vi "Module_UI_TopLevel.vi"(8 "error in (no error)":errorcluster, 10 "Wait on Module(s) (\"\": none)":string) -> (0 "error out":errorcluster)   [LabVIEW 2020, in "Module_UI_TopLevel.lvclass"]
doc: "created using\nJSMA Module Template - UI Class 0.3.0.13\nRob Humfeld - Jet Engineering\nCopyright (c) 2020, Jet Engineering"
uses:
  Module_UI_TopLevel.lvclass
  Module_UI_TopLevel.lvclass/Module_UI_TopLevel.ctl
  <userlib>/JET Engineering/JET_QSM/Code/Private/JET_QSM - Add State to Front [String API].vi
  Private/Module_UI_TopLevel_jMsgTxList STYP.ctl
  <userlib>/JET Engineering/JET_QSM/Code/Private/JET_QSM - Add State [String API].vi
  Private/Module_UI_TopLevel_jMsgRxList STYP.ctl
  Private/Module_UI_TopLevel_LocalData STYP.ctl
  <userlib>/JET Labs/JET Panel/JETPanel.lvclass
  <userlib>/JET Engineering/JSMA/Libraries/jMsg_CORE/jMsg_JSMA_ApplicationShutdown/jMsg_JSMA_ApplicationShutdown.lvclass
  <userlib>/JET Engineering/JSMA/Libraries/jModule Class/jModule.lvclass
  <userlib>/JET Engineering/JSMA Standard Messages/jMsg_Sys_UIPanelOpen/jMsg_Sys_UIPanel_Open.lvclass
  shared/IPayable/IPayable.lvclass
  shared/AAccount/AAccount.lvclass
  <userlib>/Jet Labs/JET UITable/UITable.lvclass
  shared/IInfoable/IInfoable.lvclass
  Shared/Account Information STYP.ctl
  Account Types STYP.ctl
  C:/Program Files/National Instruments/LabVIEW 2020/user.lib/JET Engineering/JSMA/Libraries/jModule Class/jModule.lvclass
  C:/projects/budget_LabVIEW/Main Codeline/Software/Code/Module_UI_TopLevel/Module_UI_TopLevel.lvclass
  shared/SimpleChecking/SimpleChecking.lvclass
  shared/SimpleSavings/SimpleSavings.lvclass
  shared/SimpleCredit/SimpleCredit.lvclass
  C:/Program Files/National Instruments/LabVIEW 2020/user.lib/JET Engineering/JSMA/Libraries/jMsg Class/jMsg.lvclass
  C:/Program Files/National Instruments/LabVIEW 2020/user.lib/JET Engineering/JSMA Standard Messages/jMsg_Sys_UIPanelOpen/jMsg_Sys_UIPanel_Open.lvclass
  C:/Program Files/National Instruments/LabVIEW 2020/user.lib/JET Engineering/JSMA/Libraries/jMsg_CORE/jMsg_JSMA_ApplicationShutdown/jMsg_JSMA_ApplicationShutdown.lvclass
  C:/projects/budget_LabVIEW/Main Codeline/Software/Code/shared/ASavings/ASavings.lvclass
  C:/projects/budget_LabVIEW/Main Codeline/Software/Code/shared/AInterestAccount/AInterestAccount.lvclass
  C:/projects/budget_LabVIEW/Main Codeline/Software/Code/shared/AAccount/AAccount.lvclass
  C:/projects/budget_LabVIEW/Main Codeline/Software/Code/shared/IInfoable/IInfoable.lvclass
  C:/projects/budget_LabVIEW/Main Codeline/Software/Code/shared/IInterest/IInterest.lvclass
  C:/projects/budget_LabVIEW/Main Codeline/Software/Code/Shared/IDepositable/IDepositable.lvclass
  C:/projects/budget_LabVIEW/Main Codeline/Software/Code/shared/IWithdrawable/IWithdrawable.lvclass
  C:/projects/budget_LabVIEW/Main Codeline/Software/Code/shared/SimpleSavings/SimpleSavings.lvclass
  C:/projects/budget_LabVIEW/Main Codeline/Software/Code/shared/AChecking/AChecking.lvclass
  C:/projects/budget_LabVIEW/Main Codeline/Software/Code/shared/SimpleChecking/SimpleChecking.lvclass
  C:/projects/budget_LabVIEW/Main Codeline/Software/Code/shared/ACreditAccount/ACreditAccount.lvclass
  C:/projects/budget_LabVIEW/Main Codeline/Software/Code/shared/IBorrowable/IBorrowable.lvclass
  C:/projects/budget_LabVIEW/Main Codeline/Software/Code/shared/IPayable/IPayable.lvclass
  C:/projects/budget_LabVIEW/Main Codeline/Software/Code/shared/SimpleCredit/SimpleCredit.lvclass
panel:
  in  "Exit Button":bool
  in  "Expenses Button":bool
  in  "Accounts Button":bool
  in  "SubPanel":enum32{"Accounts", "Expenses", "Create Account"}(tab)
  in  "Remove Account Button":bool
  in  "Add Account Button":bool
  in  "Accounts List":i32(listbox)
  in  "Create Account Button":bool
  in  "Credit Limit Interval (s)":u32
  in  "Credit Limit":dbl
  in  "Account Type":T1
  in  "Routing Number":string
  in  "Initial Balance":dbl
  in  "Interest Interval (s)":u32
  in  "Interest Rate":dbl
  in  "Account Number":string
  out "winSizer B":string="W"
  out "winSizer A":string="W"
  out "jModule Name":string
  out "Recent states before Error (with tick counts) 2":string="0.167 sec ago: VI Initialize\n0.167 sec ago: Window Open\n0.110 sec ago: Control Update\n0.110 sec ago: Indicator Update\n0.000 sec ago: Error Handler\r\n"
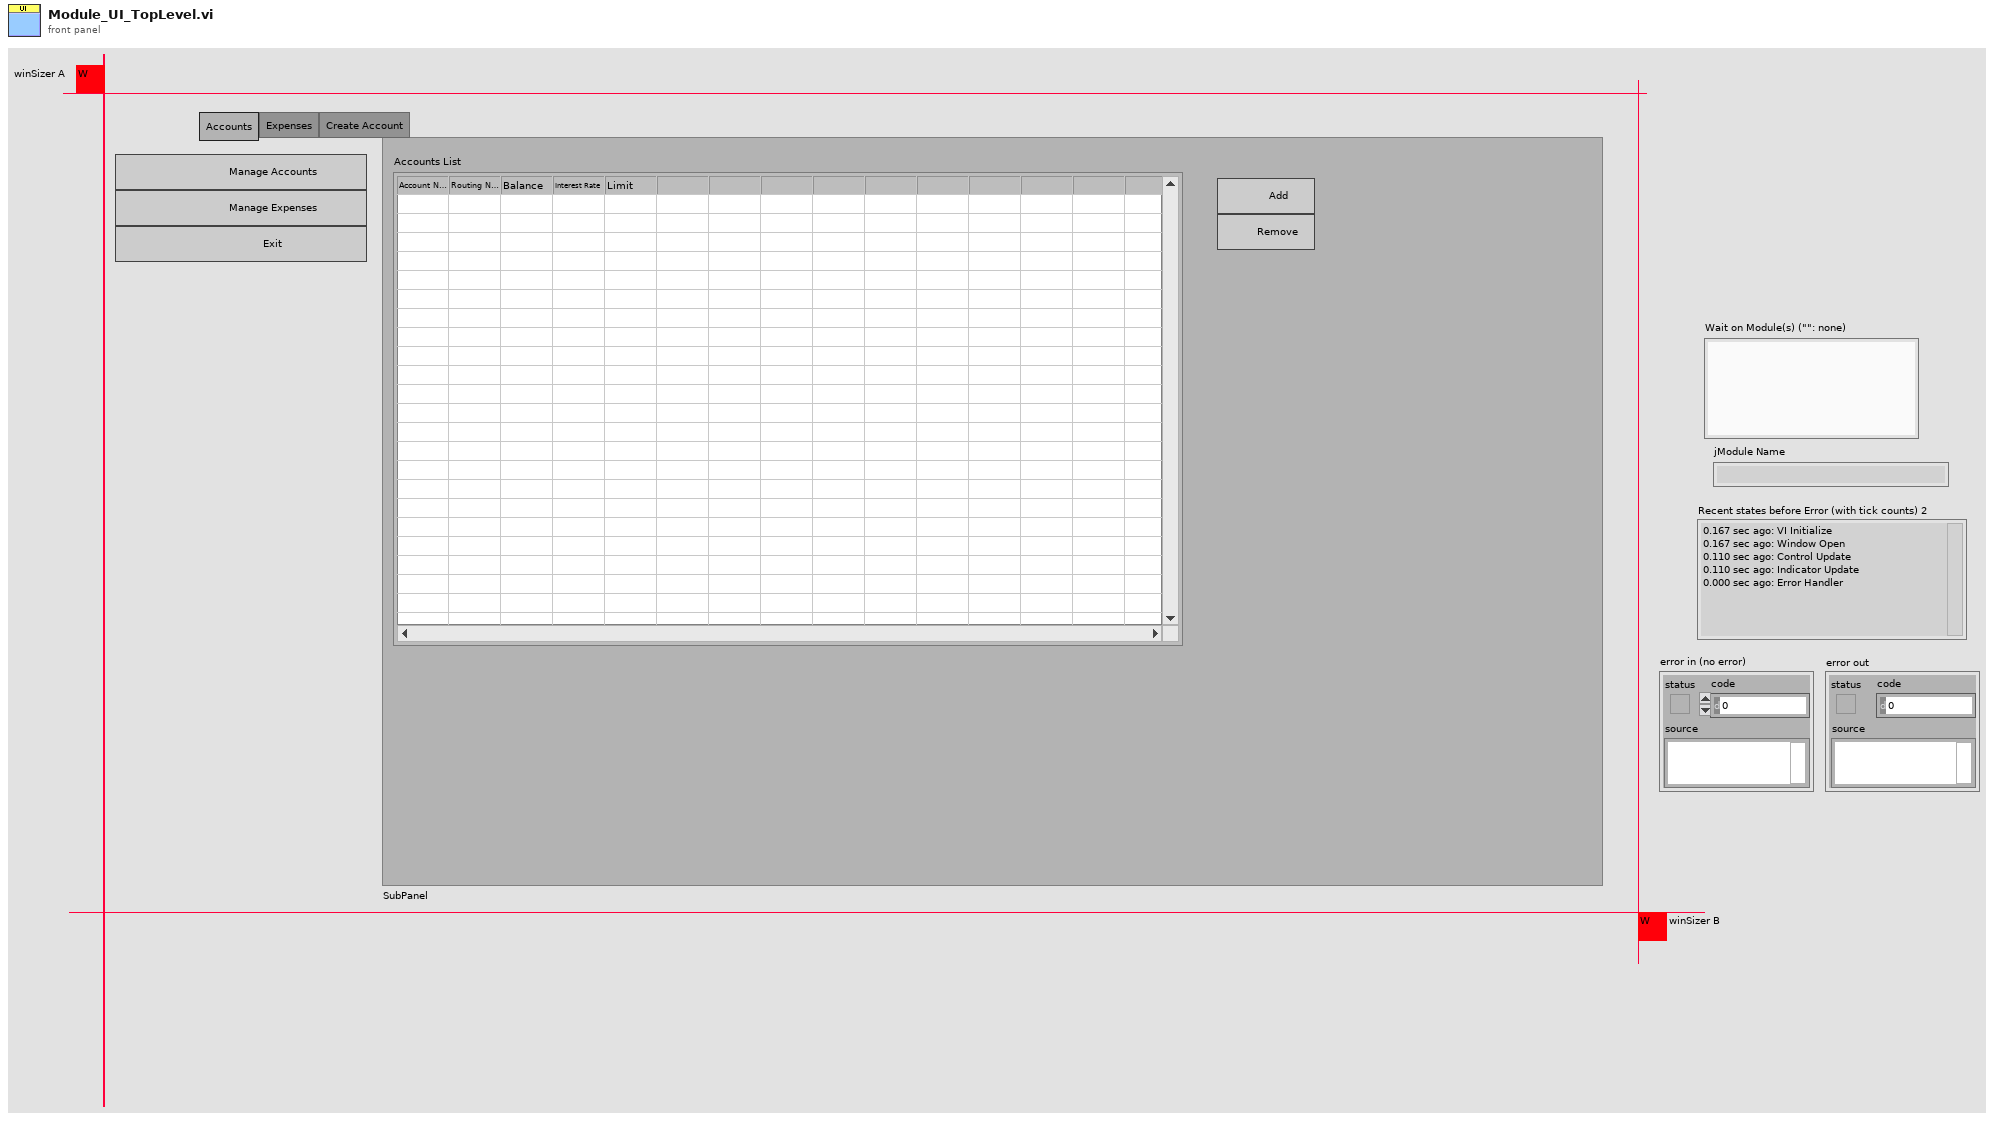
[diagram p1: front panel]
types:
  T1 = typedef "Module_UI_TopLevel.lvclass/Account Types STYP.ctl" = enum16{"Savings", "Checking", "Credit"}
  T2 = typedef "Module_UI_TopLevel.lvclass/Module_UI_TopLevel_LocalData STYP.ctl" = cluster{"VI":cluster{"error":errorcluster, "isExiting?":bool}, "UI":cluster{"Expenses":refnum<class "UITable.lvclass">, "Accounts Page":cluster{"Accounts":refnum<class "UITable.lvclass">, "Account Information":T3, "Interest Interval":u32, "Account Type":T1, "Credit Interval":u32}}, "Accounts":cluster{"Accounts":refnum<class "AAccount.lvclass">[]}, "Expenses":cluster{"Expenses":refnum<class "IPayable.lvclass">[]}}
  T3 = typedef "IInfoable.lvclass/Account Information STYP.ctl" = cluster{"Account Number":string, "Routing Number":string, "Balance":dbl, "Interest Rate":dbl, "Limit":dbl}
  T4 = typedef "Module_UI_TopLevel.lvclass/Module_UI_TopLevel_jMsgTxList STYP.ctl" = cluster{"jMsg_JSMA_ApplicationShutdown":refnum<class "jMsg_JSMA_ApplicationShutdown.lvclass">}
  T5 = typedef "Module_UI_TopLevel.lvclass/Module_UI_TopLevel_jMsgRxList STYP.ctl" = cluster{"jMsg_Sys_UIPanel_Open":refnum<class "jMsg_Sys_UIPanel_Open.lvclass">}
  T6 = typedef "JET_QSM_Refnum STYP.ctl" = cluster{"state":cluster{"queue":refnum<queue>, "idle":string, "error":string, "STOP":string}, "debug":cluster{"enabled?":bool, "queue":refnum<queue>}, "Invalid.option":T7, "QSM.Name":string}
  T7 = typedef "JET_QSM_InvalidOption STYP.ctl" = enum16{"Ignore", "Dialog", "Error"}
  T8 = typedef "JET_QSM_Element STYP.ctl" = cluster{"state":string, "data":variant, "comment":string}
  T9 = enum8{"Enabled", "Disabled", "Disabled and Grayed Out"}
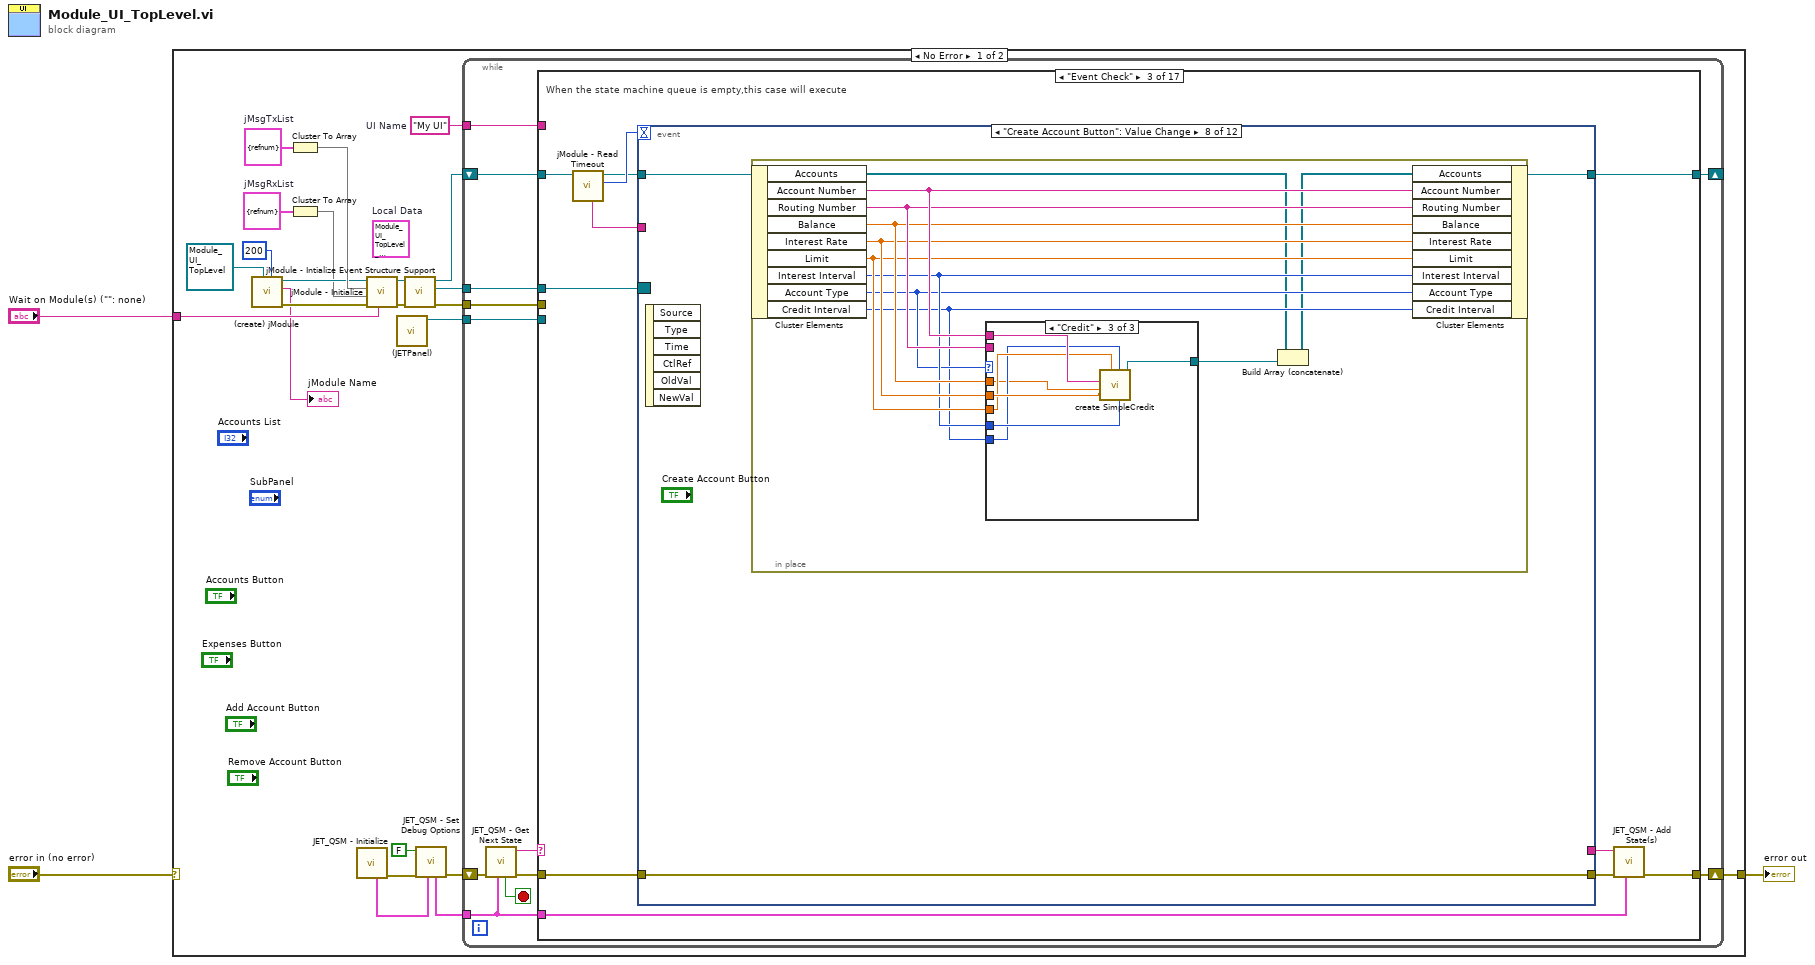
[diagram p0: block diagram]
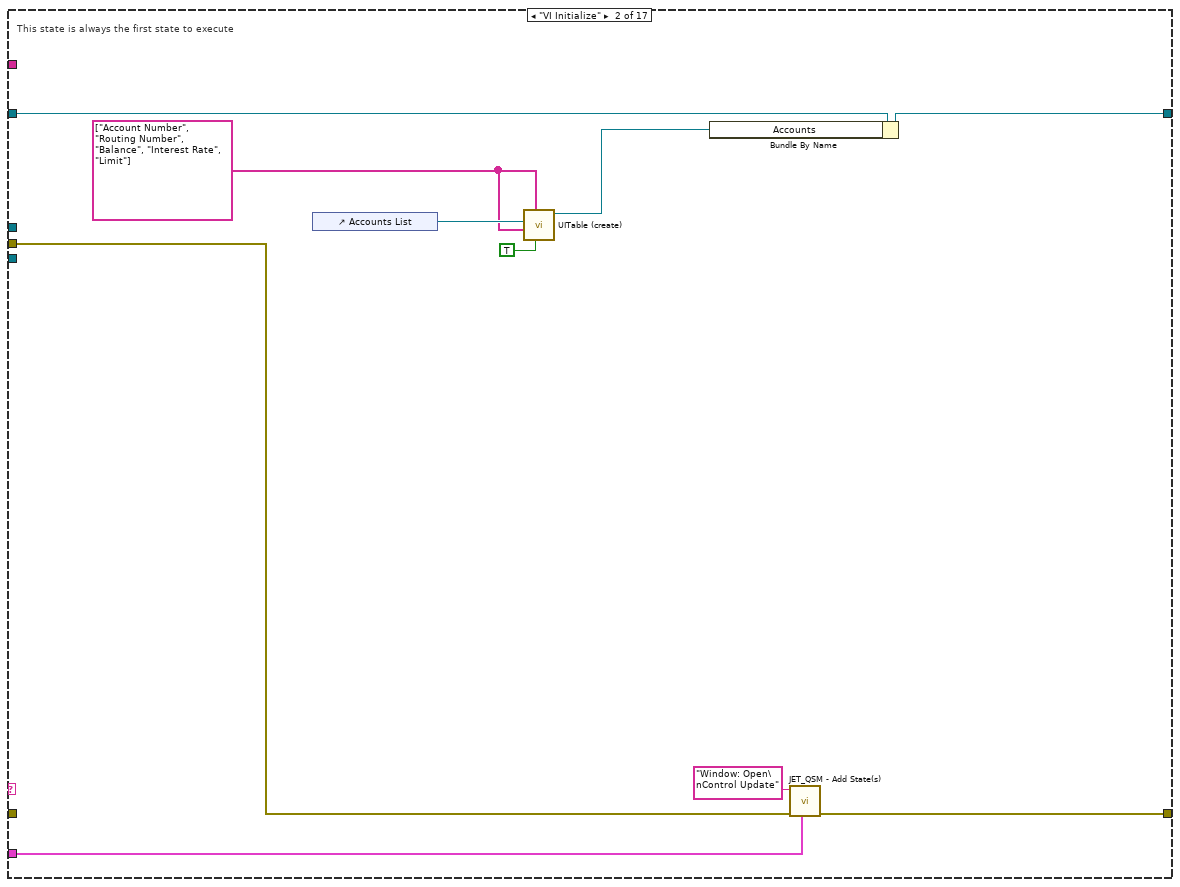
[diagram p3: hidden frame]
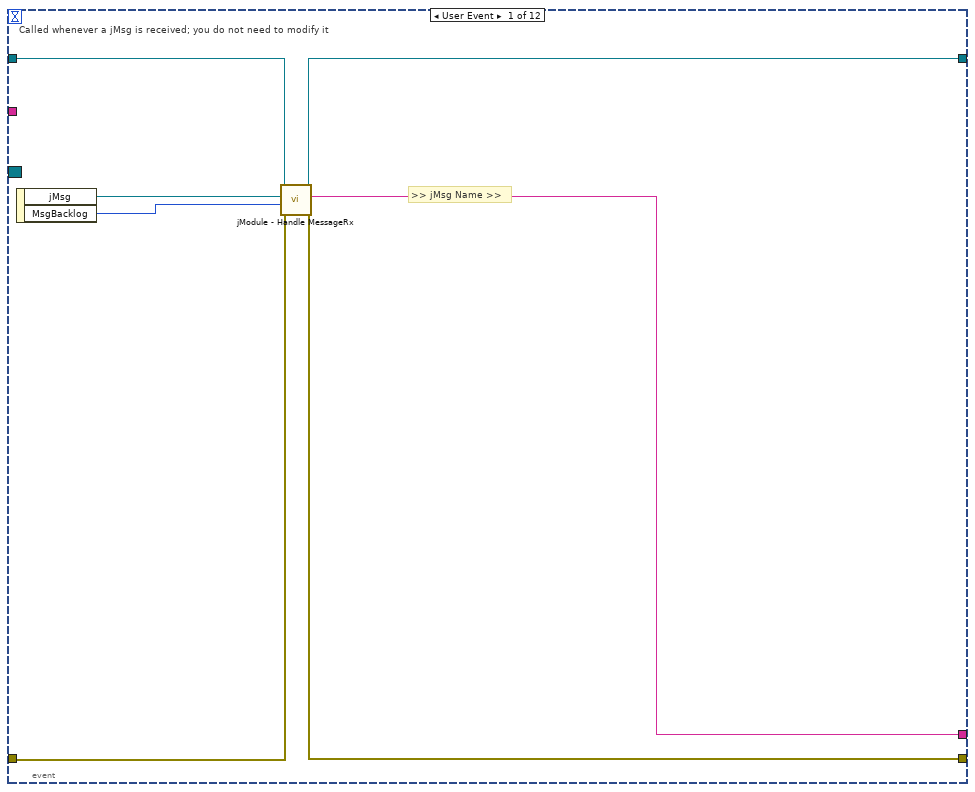
[diagram p4: hidden frame]
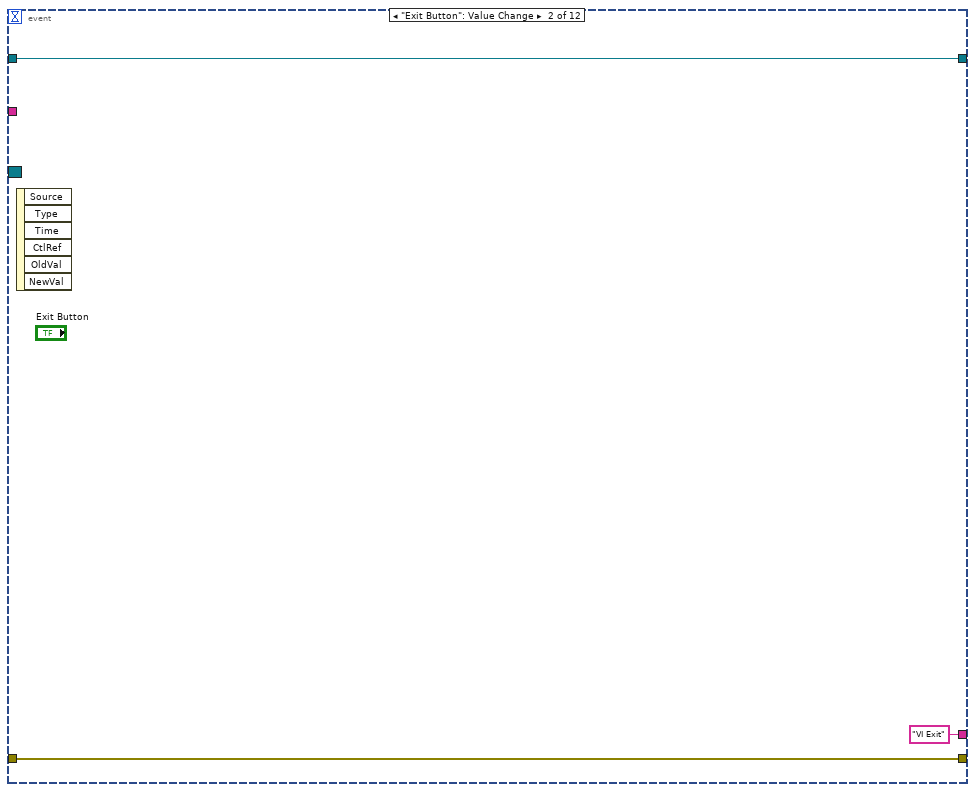
[diagram p5: hidden frame]
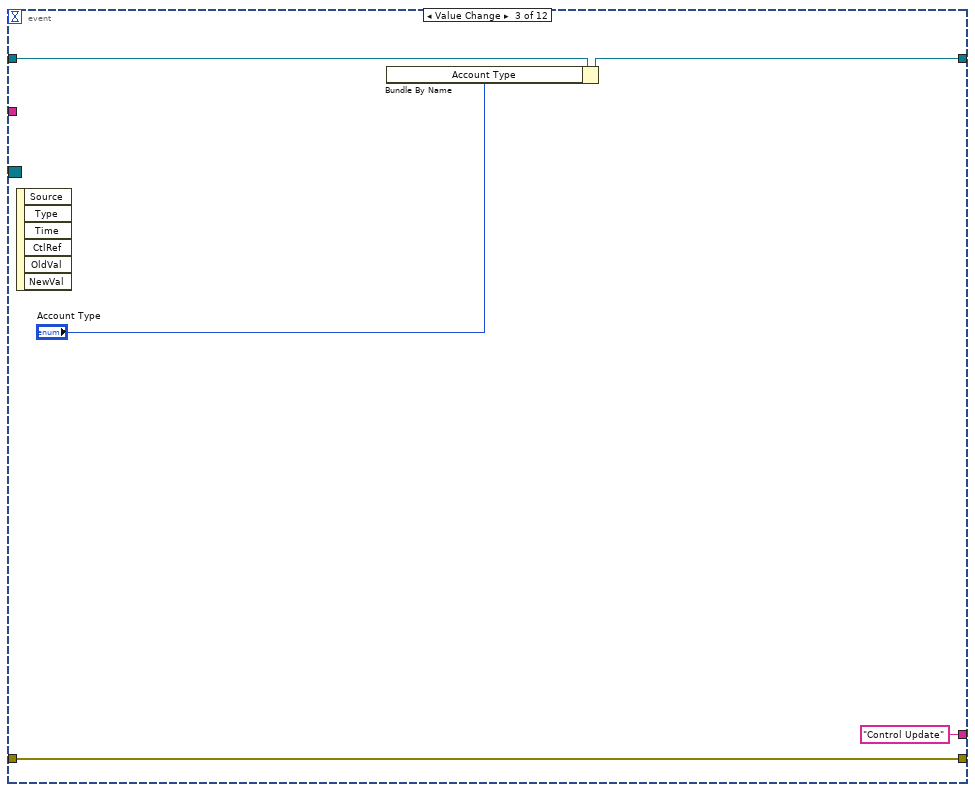
[diagram p6: hidden frame]
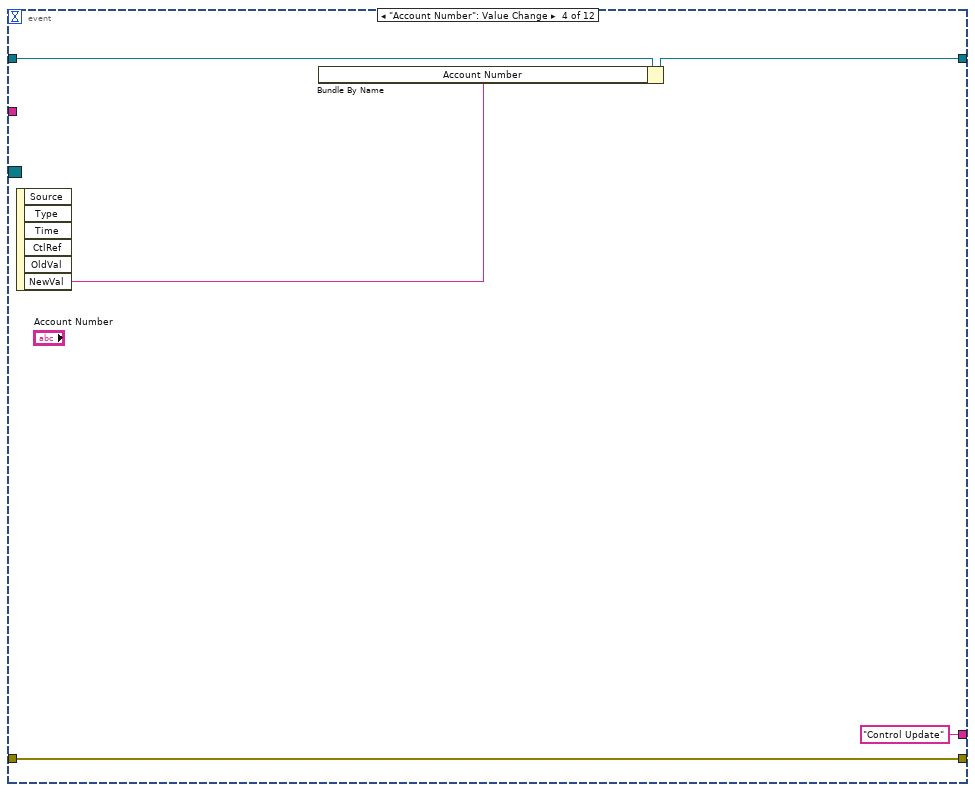
[diagram p7: hidden frame]
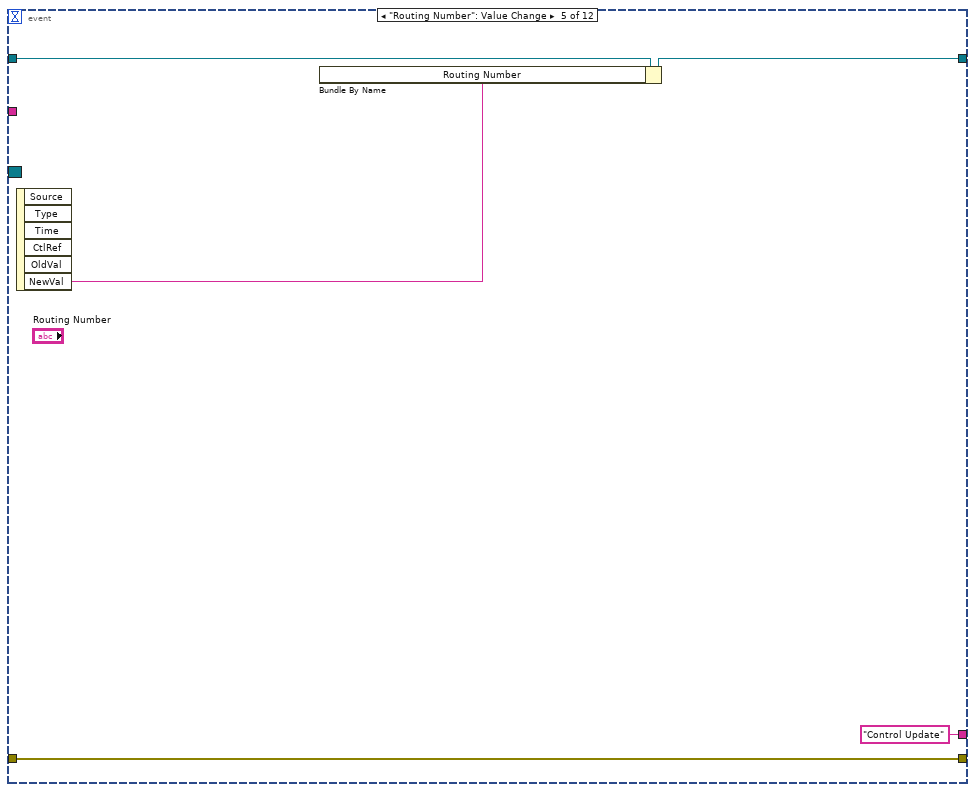
[diagram p8: hidden frame]
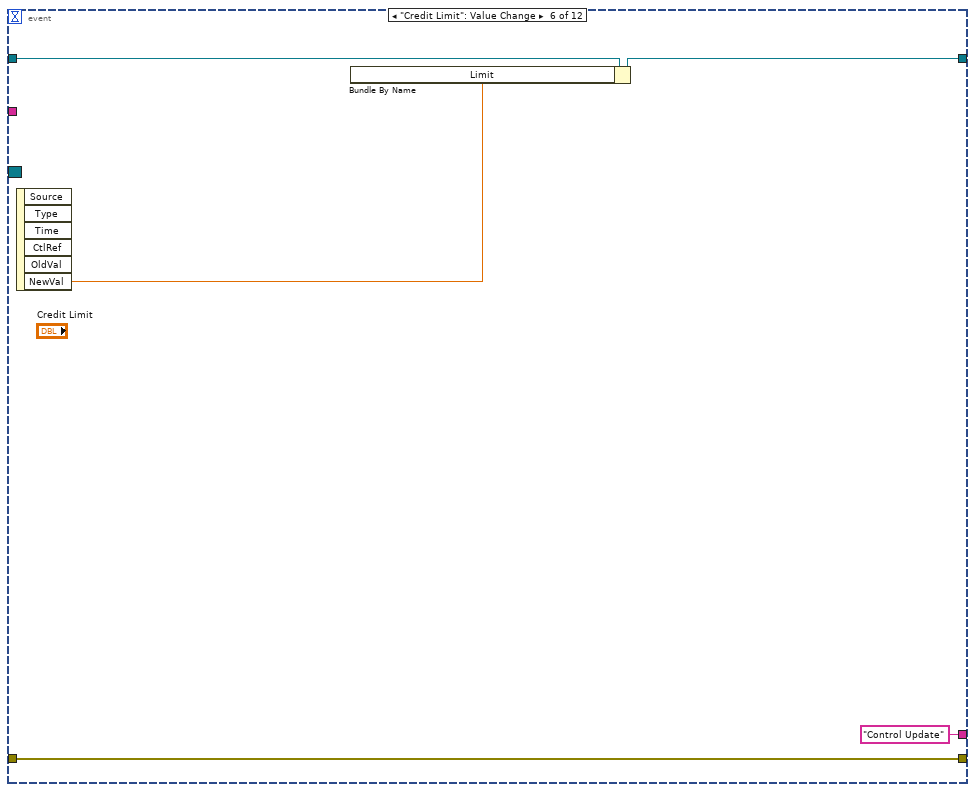
[diagram p9: hidden frame]
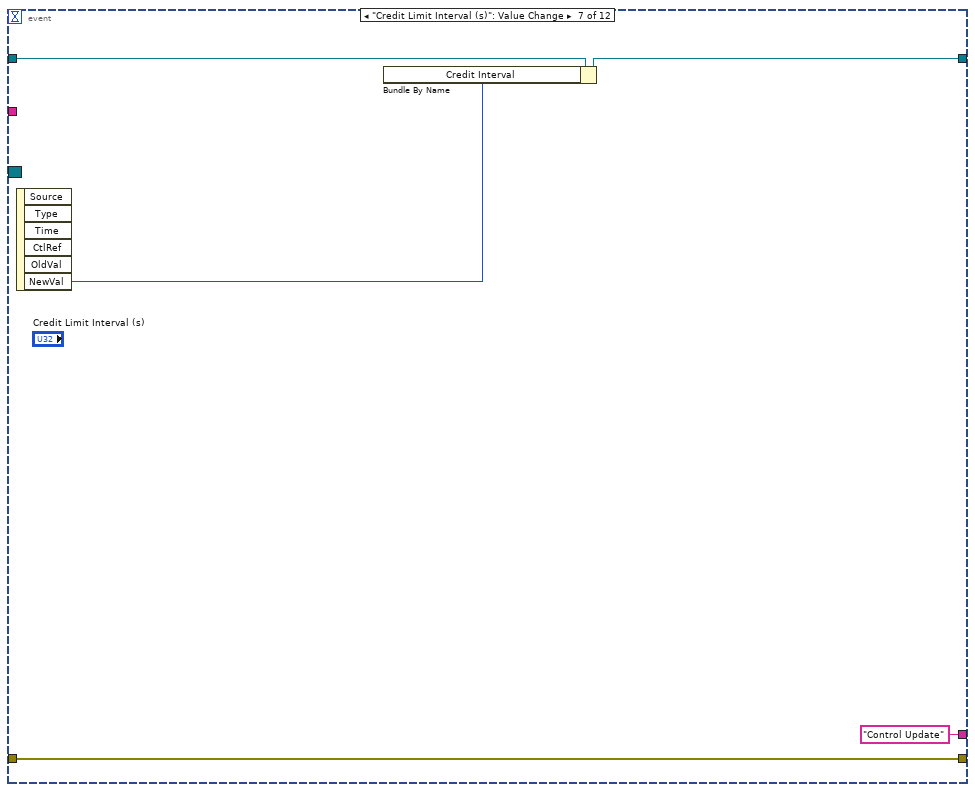
[diagram p10: hidden frame]
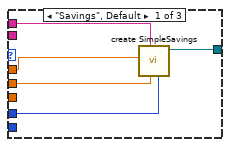
[diagram p11: hidden frame]
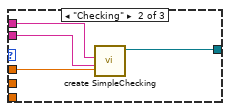
[diagram p12: hidden frame]
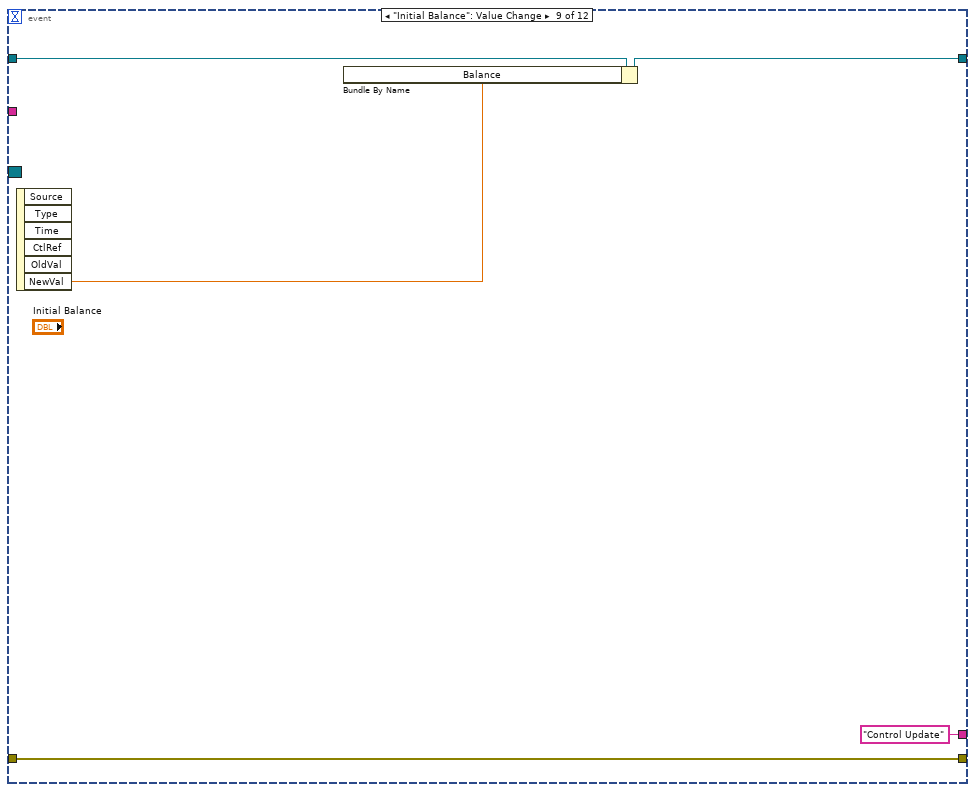
[diagram p13: hidden frame]
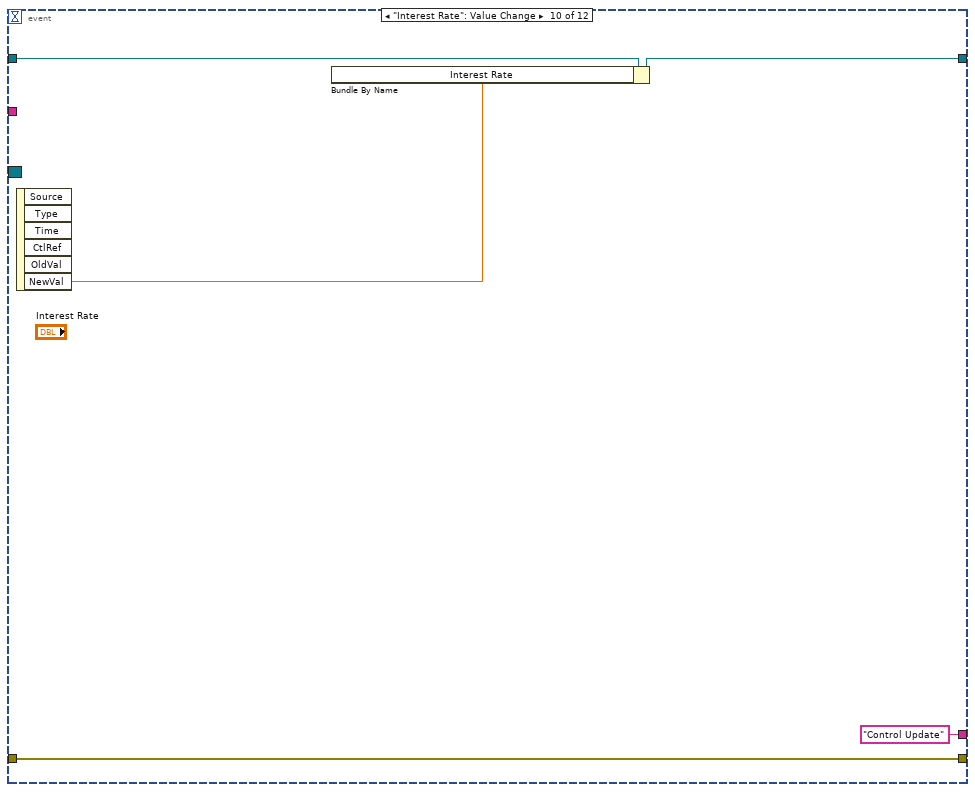
[diagram p14: hidden frame]
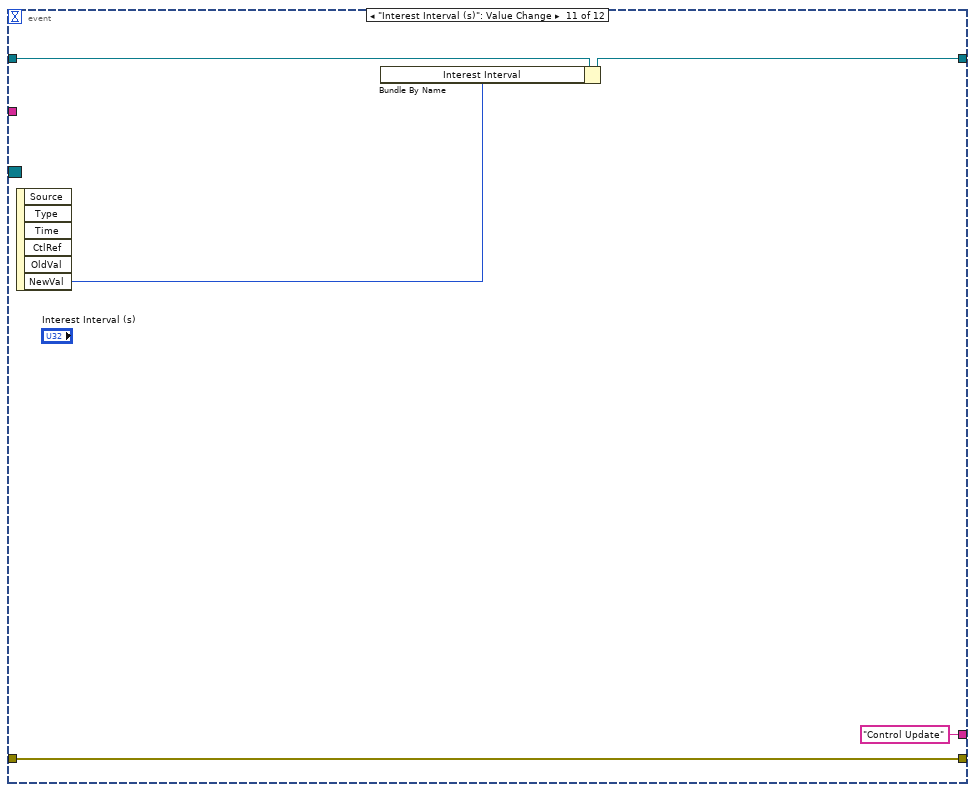
[diagram p15: hidden frame]
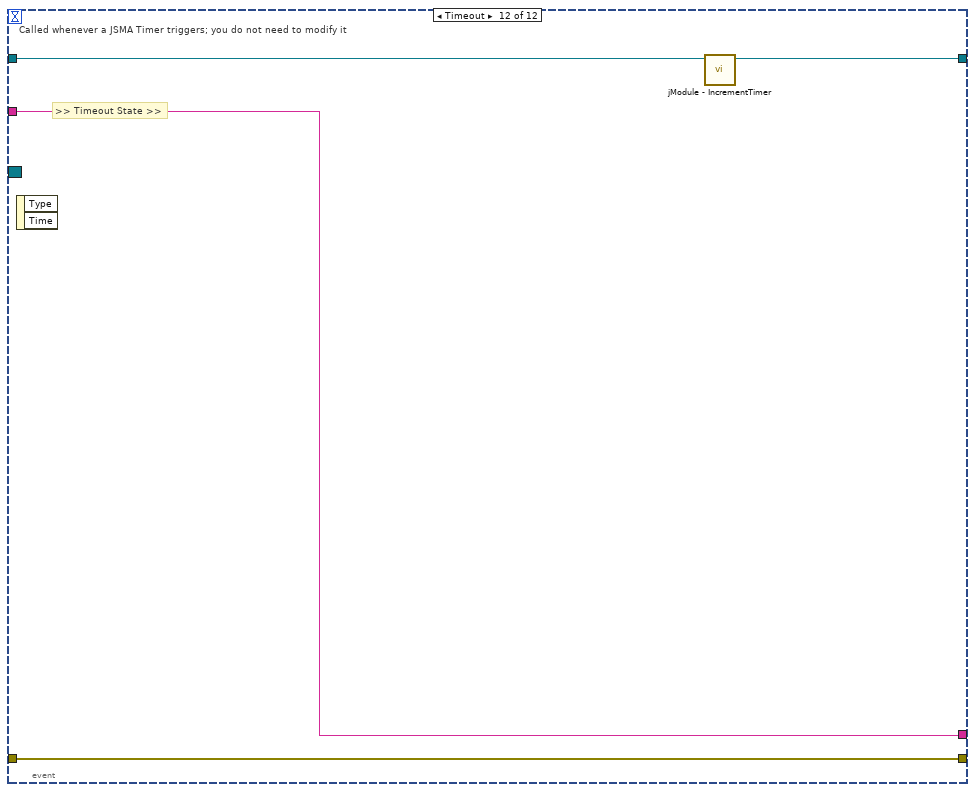
[diagram p16: hidden frame]
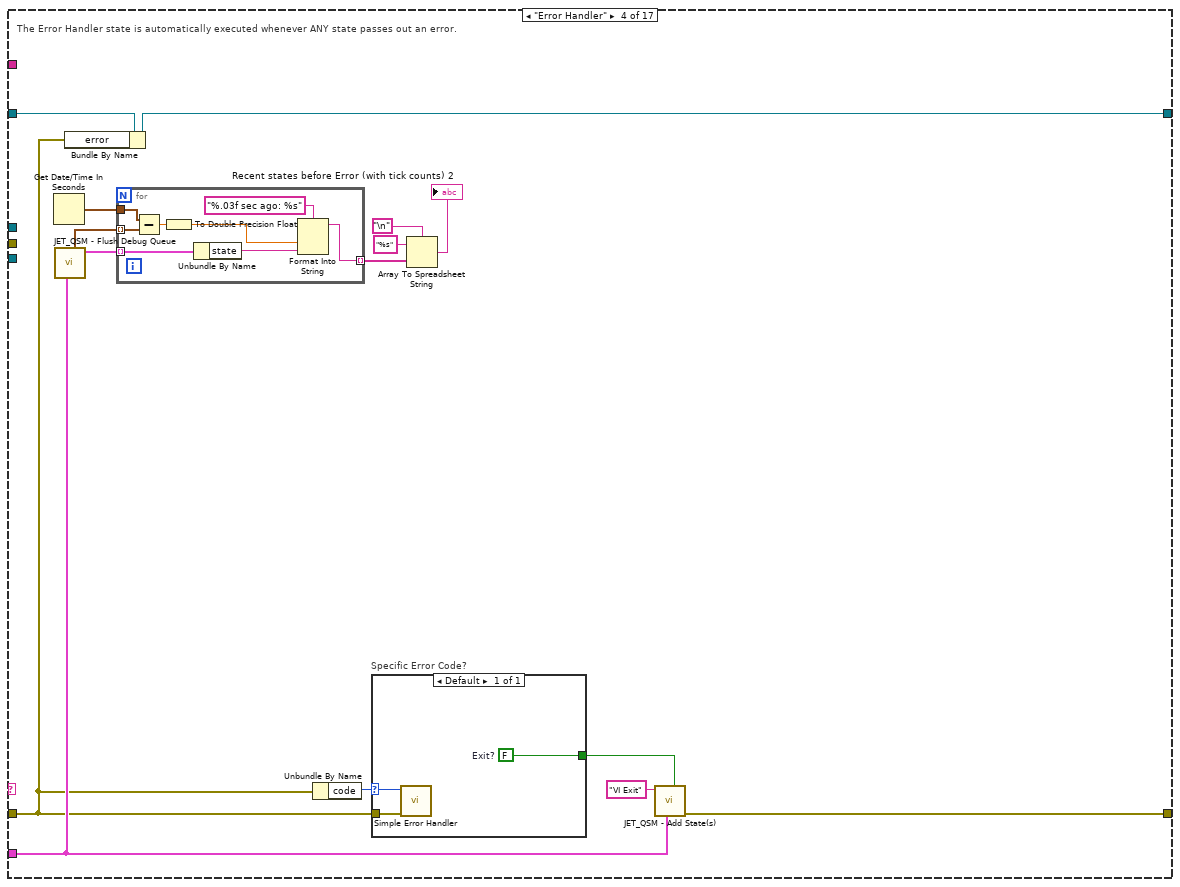
[diagram p17: hidden frame]
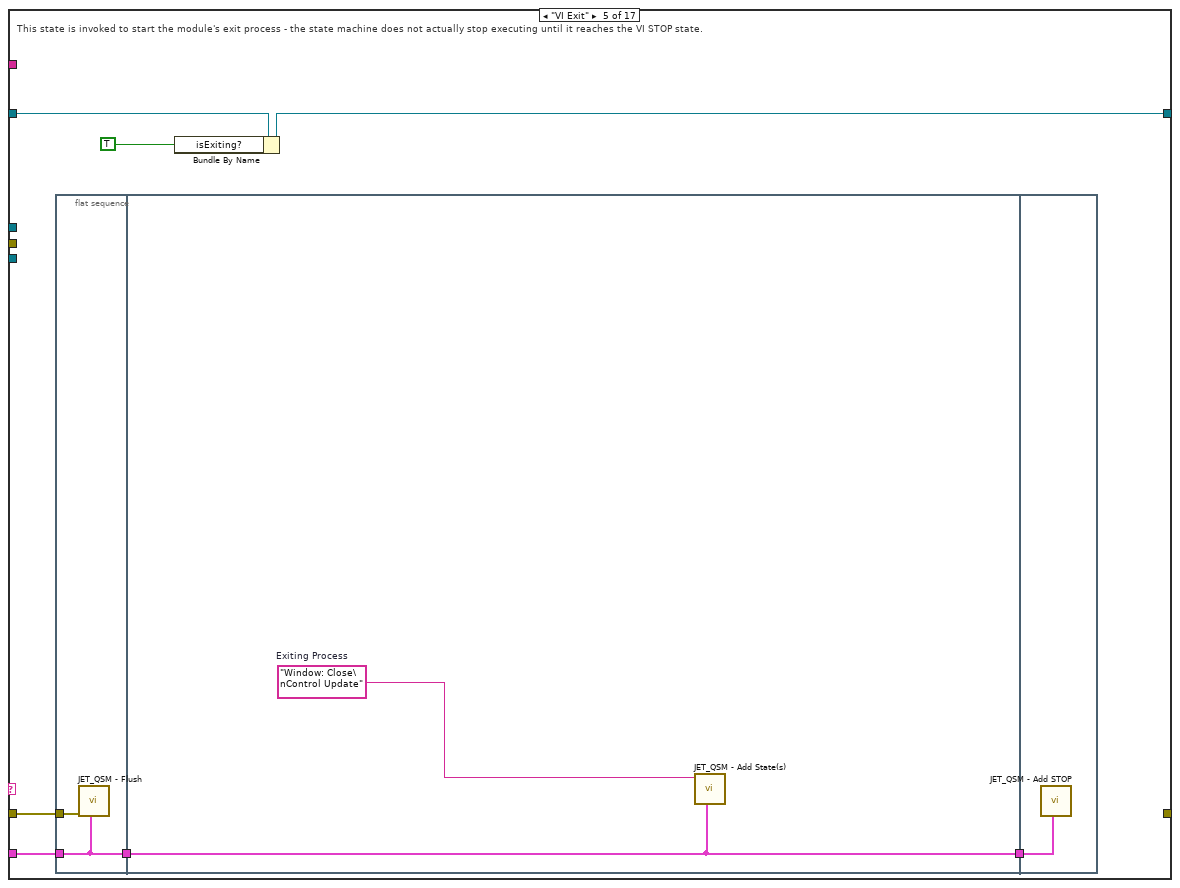
[diagram p18: hidden frame]
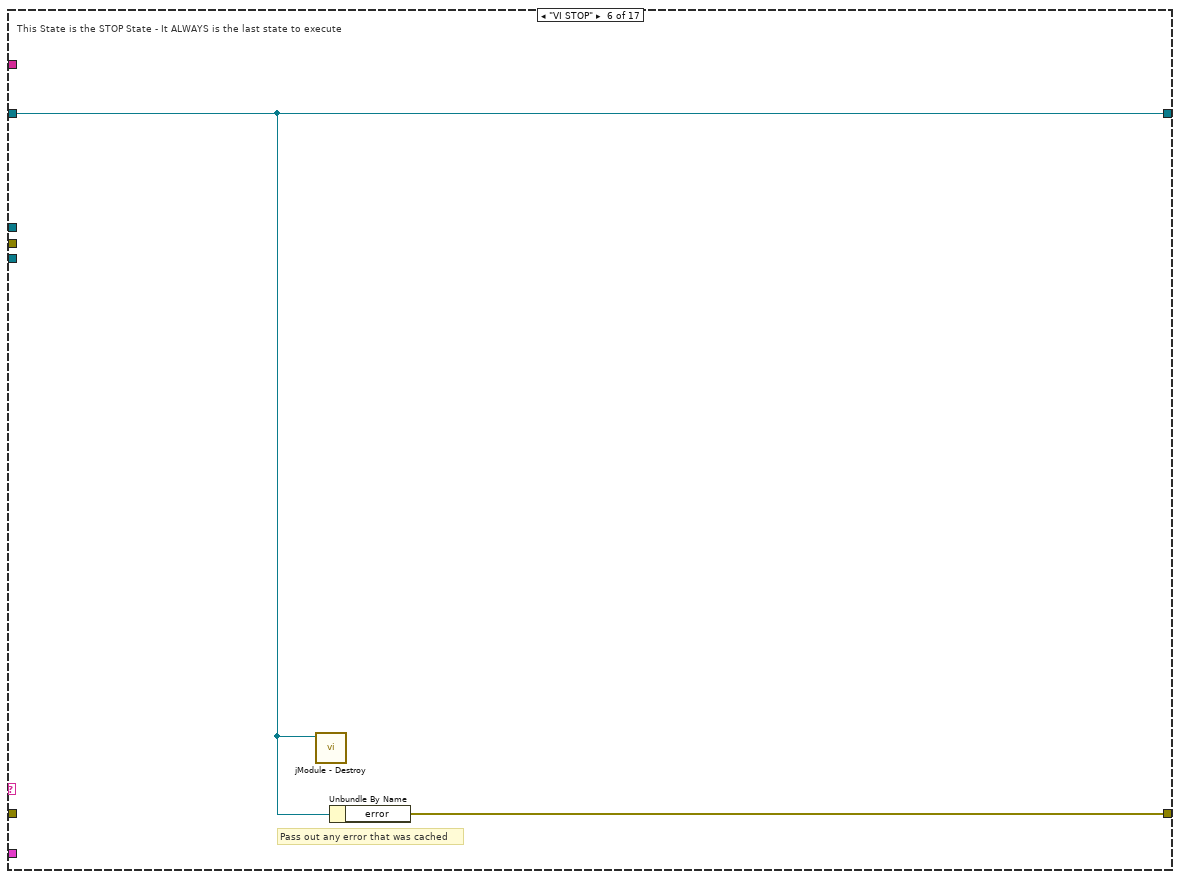
[diagram p19: hidden frame]
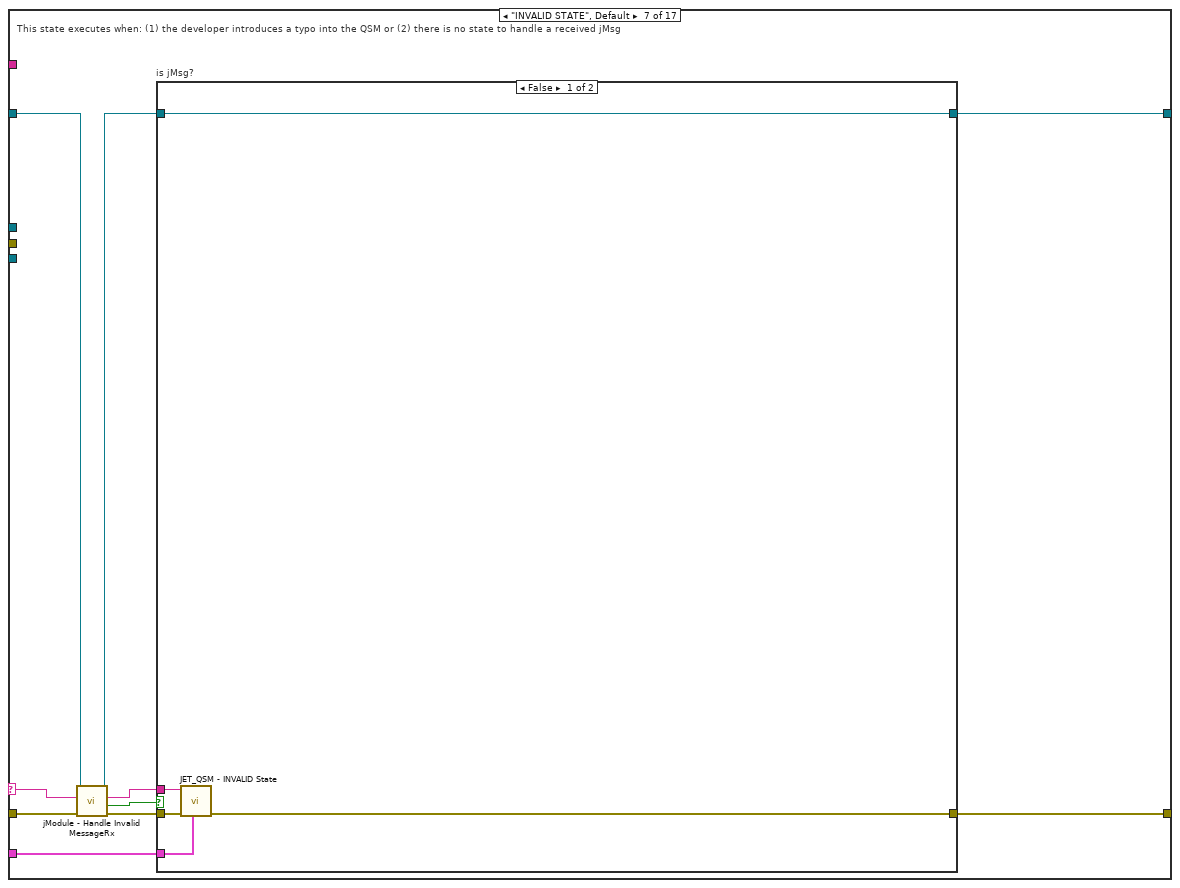
[diagram p20: hidden frame]
diagram:
  n1 = case shown="No Error" "error in (no error)" {
    selector: "error in (no error)" -> [_ w279]
    tunnel: [w26 w279] -> w3
    tunnel: "Wait on Module(s) (\"\": none)" -> [w14 _]
    frame No Error {
      (unwired) T2 {"VI"={"error"={"status"=FALSE, "code"=0, "source"=""}, "isExiting?"=FALSE}, "UI"={"Expenses"=refnum, "Accounts Page"={"Accounts"=refnum, "Account Information"={"Account Number"="", "Routing Number"="", "Balance"=0.0, "Interest Rate"=0.0, "Limit"=0.0}, "Interest Interval"=0, "Account Type"=enum."Savings", "Credit Interval"=0}}, "Accounts"={"Accounts"=[]}, "Expenses"={"Expenses"=[]}}  # Local Data
      w13 = T4 {"jMsg_JSMA_ApplicationShutdown"=refnum}  # jMsgTxList
      w12 = T5 {"jMsg_Sys_UIPanel_Open"=refnum}  # jMsgRxList
      w16 = "My UI"  # UI Name
      n2 = call <userlib>:"(create) jModule.vi"("Max Queue size (50)"=200, "jModule Child class"=refnum<class "Module_UI_TopLevel.lvclass"> refnum ("Module_UI_SystemEventLog.lvclass")) -> ("error out"=w8:errorcluster, "jModule Name"=→"jModule Name":string, "jModule"=w9:refnum<class "Module_UI_TopLevel.lvclass">)  [unwired: 6 in, 1 out]
      n3 = Cluster To Array(cluster=w13) -> (array=w20:refnum<class "jMsg_JSMA_ApplicationShutdown.lvclass">[])
      n4 = Cluster To Array(cluster=w12) -> (array=w4:refnum<class "jMsg_Sys_UIPanel_Open.lvclass">[])
      n5 = call <userlib>:"JET_QSM - Initialize.vi"() -> ("error out"=w21:errorcluster, "Jet_QSM refnum"=w24:T6)  [unwired: 10 in]
      n6 = call-dynamic "jModule - Initialize.vi"("Wait on Module(s) (\"\": none)"=w14, "error in (no error)"=w8, "jMsgRxList"=w4, "jMsgTxList"=w20, "jModule"=w9) -> ("error out"=w19:errorcluster, "jModule"=w18:refnum<class "Module_UI_TopLevel.lvclass">)  [unwired: 5 in]
      n7 = call <userlib>:"(JETPanel).vi"() -> ("JETPanel"=w6:refnum<class "JETPanel.lvclass">)  [unwired: 8 in, 3 out]
      n8 = call <userlib>:"jModule - Intialize Event Structure Support.vi"("error in (no error)"=w19, "jModule"=w18) -> ("error out"=w15:errorcluster, "Event Registration Refnum"=w17:refnum<event-registration>, "jModule"=w11:refnum<class "Module_UI_TopLevel.lvclass">)  [unwired: 6 in, 1 out]
      n9 = call <userlib>:"JET_QSM - Set Debug Options.vi"("Jet_QSM refnum"=w24, "error in (no error)"=w21, "debug.enabled? (F)"=FALSE) -> ("error out"=w22:errorcluster, "Jet_QSM ref"=w23:T6)  [unwired: 7 in]
      n10 = while {
        tunnel: w23 -> [w34]
        shift-right: [w32] -> _
        shift-left: w11 -> [w33]
        shift-right: [w31] -> w26
        shift-left: w22 -> [w38]
        tunnel: w15 -> [w30]
        tunnel: w17 -> [w29]
        tunnel: w16 -> [w28]
        tunnel: w6 -> [w27]
        stop <- w35 stop-if-true
        n11 = call <userlib>:"JET_QSM - Get Next State.vi"("Jet_QSM refnum"=w34, "error in (no error)"=w38) -> ("error out"=w37:errorcluster, "state"=w36:string, "Stop Loop?"=w35:bool)  [unwired: 5 in, 2 out]
        n12 = case shown="\"Event Check\"" w36 {
          selector: w36 -> [_ _ _ _ _ _ w188 _ _ _ _ _ _ _ _ _ _]
          tunnel: w37 -> [w39 _ w61 w148 w178 _ w190 w203 w210 w214 w219 w227 w231 w237 w243 w270 w278]
          tunnel: w34 -> [_ w50 w60 w152 w177 _ w194 _ w213 w218 _ _ _ w238 w244 w271 _]
          tunnel: w33 -> [w40 w47 w52 w147 w175 w184 w192 w204 w207 w215 w220 w226 w232 w241 w247 w266 w277]
          tunnel: [w40 w45 w56 w146 w174 w184 w193 w204 w206 w215 w220 w222 w232 w241 w247 w267 w277] -> w32
          tunnel: [w39 w49 w58 w153 _ w185 w195 w203 w212 w217 w219 w227 w231 w236 w242 w269 w278] -> w31
          tunnel: w30 -> [_ w48 _ _ _ _ _ _ _ _ _ _ _ _ _ _ _]
          tunnel: w29 -> [_ _ w55 _ _ _ _ _ _ _ _ _ _ _ _ _ _]
          tunnel: w28 -> [_ _ _ _ _ _ _ _ w209 _ _ _ _ w233 _ _ _]
          tunnel: w27 -> [_ _ _ _ _ _ _ _ _ _ _ _ _ w240 w246 _ _]
          frame "------ Standard States ------" {
            # "Standard States are required states for a JET_QSM State Machine\n\nTheir names may be changed; see the JET QSM Initialize function to specify the new names"
            # "This is a section header; the state is never expected to execute"
          }
          frame "VI Initialize" {
            w41 = string[] ["Account Number", "Routing Number", "Balance", "Interest Rate", "Limit"] ("TableColumnHeaderLabel[]")
            # "This state is always the first state to execute"
            n13 = control-ref of="Accounts List"() -> (w43:refnum<vi>)
            n14 = call <userlib>:"UITable (create).vi"("Set Column Headers? (F)"=TRUE, "TableColumnHeaderLabel[]"=w41, "DataColumnID[]"=w41, "MCListbox.refnum"=w43) -> ("UITable"=w44:refnum<class "UITable.lvclass">)  [unwired: 6 in, 1 out]
            n15 = Bundle By Name(cluster=w47, "Accounts"=w44) -> (w45:refnum<class "Module_UI_TopLevel.lvclass">)
            n16 = call-poly <userlib>:"JET_QSM - Add State(s).vi"("Jet_QSM refnum"=w50, "error in (no error)"=w48, "state(s)"="Window: Open\nControl Update") -> ("error out"=w49:errorcluster)  [unwired: 8 in]
          }
          frame "Event Check" {
            # "When the state machine queue is empty,this case will execute"
            n17 = call <userlib>:"jModule - Read Timeout.vi"("jModule"=w52) -> ("Timeout, ms"=w54:i32, "jModule"=w51:refnum<class "Module_UI_TopLevel.lvclass">, "Timeout.State"=w53:string)  [unwired: 8 in]
            n18 = event shown="[7] \"Create Account Button\": Value Change" {
              selector: w55 -> [_ _ _ _ _ _ _ _ _ _ _ _]
              dyn-events: _ -> [_ _ _ _ _ _ _ _ _ _ _ _]
              timeout: w54 -> [_ _ _ _ _ _ _ _ _ _ _ _]
              tunnel: w61 -> [w66 w71 w76 w81 w86 w91 w96 w99 w131 w136 w141 w144]
              tunnel: [w67 "VI Exit" ("Timeout.State") "Control Update" ("Timeout.State") "Control Update" ("Timeout.State") "Control Update" ("Timeout.State") "Control Update" ("Timeout.State") "Control Update" ("Timeout.State") _ "Control Update" ("Timeout.State") "Control Update" ("Timeout.State") "Control Update" ("Timeout.State") w145] -> w59
              tunnel: [w65 w71 w76 w81 w86 w91 w96 w99 w131 w136 w141 w144] -> w57
              tunnel: w51 -> [w63 w70 w75 w80 w85 w90 w95 w98 w130 w135 w140 w143]
              tunnel: [w62 w70 w73 w78 w83 w88 w93 w97 w128 w133 w138 w142] -> w56
              tunnel: w53 -> [_ _ _ _ _ _ _ _ _ _ _ w145]
              event User Event {
                # ">> jMsg Name >>"
                # "Called whenever a jMsg is received; you do not need to modify it"
                n19 = event-data() -> ("jMsg"=w68:refnum<class "jMsg.lvclass">, "MsgBacklog"=w64:i32)  [unwired: 1 in]
                n20 = call-dynamic "jModule - Handle MessageRx.vi"("error in (no error)"=w66, "Message Backlog"=w64, "jMsg"=w68, "jModule"=w63) -> ("error out"=w65:errorcluster, "QSMState"=w67:string, "jModule"=w62:refnum<class "Module_UI_TopLevel.lvclass">)  [unwired: 4 in, 1 out]
              }
              event "Exit Button": Value Change {
                n21 = event-data() -> ()  [unwired: 1 in, 6 out]
              }
              event Value Change {
                n22 = event-data() -> ()  [unwired: 1 in, 6 out]
                n23 = Bundle By Name(cluster=w75, "Account Type"="Account Type") -> (w73:refnum<class "Module_UI_TopLevel.lvclass">)
              }
              event "Account Number": Value Change {
                n24 = event-data() -> ("NewVal"=w77:string)  [unwired: 1 in, 5 out]
                n25 = Bundle By Name(cluster=w80, "Account Number"=w77) -> (w78:refnum<class "Module_UI_TopLevel.lvclass">)
              }
              event "Routing Number": Value Change {
                n26 = event-data() -> ("NewVal"=w82:string)  [unwired: 1 in, 5 out]
                n27 = Bundle By Name(cluster=w85, "Routing Number"=w82) -> (w83:refnum<class "Module_UI_TopLevel.lvclass">)
              }
              event "Credit Limit": Value Change {
                n28 = event-data() -> ("NewVal"=w87:dbl)  [unwired: 1 in, 5 out]
                n29 = Bundle By Name(cluster=w90, "Limit"=w87) -> (w88:refnum<class "Module_UI_TopLevel.lvclass">)
              }
              event "Credit Limit Interval (s)": Value Change {
                n30 = event-data() -> ("NewVal"=w92:u32)  [unwired: 1 in, 5 out]
                n31 = Bundle By Name(cluster=w95, "Credit Interval"=w92) -> (w93:refnum<class "Module_UI_TopLevel.lvclass">)
              }
              event "Create Account Button": Value Change {
                n32 = event-data() -> ()  [unwired: 1 in, 6 out]
                n33 = in-place {
                  n34 = in-place-cluster #1(w98) -> ("Accounts"=w102:refnum<class "AAccount.lvclass">[], "Account Number"=w110:string, "Routing Number"=w109:string, "Balance"=w108:dbl, "Interest Rate"=w107:dbl, "Limit"=w106:dbl, "Interest Interval"=w105:u32, "Account Type"=w104:T1, "Credit Interval"=w103:u32)
                  n35 = case shown="\"Credit\"" w104 {
                    tunnel: w110 -> [w114 w119 w123]
                    tunnel: w109 -> [_ w118 _]
                    tunnel: w108 -> [w113 w117 w120]
                    tunnel: w107 -> [w112 _ w125]
                    tunnel: w106 -> [_ _ w122]
                    tunnel: w105 -> [w111 _ w124]
                    tunnel: w103 -> [_ _ w121]
                    tunnel: [w115 w116 w126] -> w100
                    frame "Savings", Default {
                      n36 = call "create SimpleSavings.vi"("Interest Rate Interval (s)"=w111, "Interest Rate"=w112, "Account Number"=w114, "Initial Balance"=w113) -> ("SimpleSavings out"=w115:refnum<class "SimpleSavings.lvclass">)  [unwired: 6 in, 1 out]
                    }
                    frame "Checking" {
                      n37 = call "create SimpleChecking.vi"("Inital Amount (0)"=w117, "Routing Number"=w118, "Account Number"=w119) -> ("SimpleChecking out"=w116:refnum<class "SimpleChecking.lvclass">)  [unwired: 7 in, 1 out]
                    }
                    frame "Credit" {
                      n38 = call "create SimpleCredit.vi"("Interest Rate Interval (s)"=w124, "Credit Limit Interval (s)"=w121, "Interest Rate"=w125, "Credit Limit"=w122, "Initial Balance"=w120, "Account Number"=w123) -> ("SimpleCredit out"=w126:refnum<class "SimpleCredit.lvclass">)  [unwired: 4 in, 1 out]
                    }
                  }
                  n39 = Build Array (concatenate)(w102, w100) -> (w101:refnum<class "AAccount.lvclass">[])
                  n40 = in-place-cluster #1("Accounts"=w101, "Account Number"=w110, "Routing Number"=w109, "Balance"=w108, "Interest Rate"=w107, "Limit"=w106, "Interest Interval"=w105, "Account Type"=w104, "Credit Interval"=w103) -> (w97:refnum<class "Module_UI_TopLevel.lvclass">)
                }
              }
              event "Initial Balance": Value Change {
                n41 = event-data() -> ("NewVal"=w127:dbl)  [unwired: 1 in, 5 out]
                n42 = Bundle By Name(cluster=w130, "Balance"=w127) -> (w128:refnum<class "Module_UI_TopLevel.lvclass">)
              }
              event "Interest Rate": Value Change {
                n43 = event-data() -> ("NewVal"=w132:dbl)  [unwired: 1 in, 5 out]
                n44 = Bundle By Name(cluster=w135, "Interest Rate"=w132) -> (w133:refnum<class "Module_UI_TopLevel.lvclass">)
              }
              event "Interest Interval (s)": Value Change {
                n45 = event-data() -> ("NewVal"=w137:u32)  [unwired: 1 in, 5 out]
                n46 = Bundle By Name(cluster=w140, "Interest Interval"=w137) -> (w138:refnum<class "Module_UI_TopLevel.lvclass">)
              }
              event Timeout {
                # ">> Timeout State >>"
                # "Called whenever a JSMA Timer triggers; you do not need to modify it"
                n47 = event-data() -> ()  [unwired: 1 in, 2 out]
                n48 = call <userlib>:"jModule - IncrementTimer.vi"("jModule"=w143) -> ("jModule"=w142:refnum<class "Module_UI_TopLevel.lvclass">)  [unwired: 10 in]
              }
            }
            n49 = call-poly <userlib>:"JET_QSM - Add State(s).vi"("Jet_QSM refnum"=w60, "error in (no error)"=w57, "state(s)"=w59) -> ("error out"=w58:errorcluster)  [unwired: 8 in]
          }
          frame "Error Handler" {
            # "The Error Handler state is automatically executed whenever ANY state passes out an error."
            n50 = Get Date/Time In Seconds() -> (seconds since 1Jan1904=w156:timestamp)
            n51 = call <userlib>:"JET_QSM - Flush Debug Queue.vi"("Jet_QSM refnum"=w152) -> ("QSM Elements"=w154:T8[], "Timestamps"=w155:timestamp[])  [unwired: 8 in, 1 out]
            n52 = Bundle By Name(cluster=w147, "error"=w148) -> (w146:refnum<class "Module_UI_TopLevel.lvclass">)
            n53 = for {
              tunnel: w154 -> [w168] mode=indexing
              tunnel: [w166] -> w158 mode=indexing
              tunnel: w156 -> [w163]
              tunnel: w155 -> [w164] mode=indexing
              n54 = Subtract(x=w163, y=w164) -> (x-y=w162:dbl)
              n55 = To Double Precision Float(number=w162) -> (double precision float=w161:dbl)
              n56 = Unbundle By Name(w168) -> ("state"=w167:string)
              n57 = Format Into String(format string="%.03f sec ago: %s", w161, w167) -> (resulting string=w166:string)  [unwired: 2 in, 1 out]
            }
            n58 = Unbundle By Name(w148) -> ("code"=w149:i32)
            n59 = case "Specific Error Code?" shown="Default" w149 {
              selector: w149 -> [w170]
              tunnel: [w171] -> w150
              tunnel: w148 -> [w169]
              frame Default {
                w171 = FALSE  # Exit?
                n60 = call <vilib>:"Simple Error Handler.vi"("error code (no error:0)"=w170, "error in (no error)"=w169) -> ()  [unwired: 3 in, 5 out]
              }
            }
            n61 = Array To Spreadsheet String(delimiter (Tab)="\n", array=w158, 3:"%s" ("format string")) -> (spreadsheet string=→"Recent states before Error (with tick counts) 2":string)
            n62 = call-poly <userlib>:"JET_QSM - Add State(s).vi"("act? (T)"=w150, "Jet_QSM refnum"=w152, "state(s)"="VI Exit") -> ("error out"=w153:errorcluster)  [unwired: 8 in]
          }
          frame "VI Exit" {
            # "This state is invoked to start the module's exit process - the state machine does not actually stop executing until it reaches the VI STOP state."
            n63 = flat-sequence {
              tunnel: w178 -> [w180]
              tunnel: w177 -> [w179]
              tunnel: [w179] -> w176
              tunnel: w176 -> [w182]
              tunnel: [w182] -> w172
              tunnel: w172 -> [w183]
              frame #0 {
                n64 = call <userlib>:"JET_QSM - Flush.vi"("Jet_QSM ref"=w179, "error in (no error)"=w180) -> ()  [unwired: 8 in, 2 out]
              }
              frame #1 {
                w181 = "Window: Close\nControl Update"  # Exiting Process
                n65 = call-poly <userlib>:"JET_QSM - Add State(s).vi"("Jet_QSM refnum"=w182, "state(s)"=w181) -> ()  [unwired: 9 in, 1 out]
              }
              frame #2 {
                n66 = call <userlib>:"JET_QSM - Add STOP.vi"("Jet_QSM refnum"=w183) -> ()  [unwired: 10 in, 1 out]
              }
            }
            n67 = Bundle By Name(cluster=w175, "isExiting?"=TRUE ("VI.isExiting?")) -> (w174:refnum<class "Module_UI_TopLevel.lvclass">)
          }
          frame "VI STOP" {
            # "Pass out any error that was cached"
            # "This State is the STOP State - It ALWAYS is the last state to execute"
            n68 = call-dynamic "jModule - Destroy.vi"("jModule"=w184) -> ()  [unwired: 10 in, 1 out]
            n69 = Unbundle By Name(w184) -> ("error"=w185:errorcluster)
          }
          frame "INVALID STATE", Default {
            # "This state executes when: (1) the developer introduces a typo into the QSM or (2) there is no state to handle a received jMsg"
            n70 = call-dynamic "jModule - Handle Invalid MessageRx.vi"("error in (no error)"=w190, "Invalid State"=w188, "jModule"=w192) -> ("error out"=w189:errorcluster, "is jMsg State?"=w186:bool, "Invalid State"=w187:string, "jModule"=w191:refnum<class "Module_UI_TopLevel.lvclass">)  [unwired: 5 in]
            n71 = case "is jMsg?" shown="False" w186 {
              tunnel: [w200 w202] -> w195
              tunnel: w189 -> [w199 w202]
              tunnel: w194 -> [w198 _]
              tunnel: w191 -> [w197 w201]
              tunnel: [w197 w201] -> w193
              tunnel: w187 -> [w196 _]
              frame False {
                n72 = call <userlib>:"JET_QSM - INVALID State.vi"("Jet_QSM refnum"=w198, "error in (no error)"=w199, "state"=w196) -> ("error out"=w200:errorcluster)  [unwired: 8 in]
              }
              frame True {
              }
            }
          }
          frame "------ jMsg  ------" {
            # "This is a section header; the state is never expected to execute"
          }
          frame "jMsg_Sys_UIPanel_Open" {
            # "This is a JSMA Standard jMsg"
            n73 = call <userlib>:"jMsg_Sys_UIPanel_Open - Rx Read.vi"("jModule"=w207) -> ("UI Name"=w205:string, "jModule"=w206:refnum<class "Module_UI_TopLevel.lvclass">)  [unwired: 6 in, 3 out]
            n74 = Equal?(x=w209, y=w205) -> (x = y?=w208:bool)
            n75 = call-poly <userlib>:"JET_QSM - Add State(s).vi"("act? (T)"=w208, "Jet_QSM refnum"=w213, "error in (no error)"=w210, "state(s)"="Window: Open") -> ("error out"=w212:errorcluster)  [unwired: 7 in]
          }
          frame "jMsg_JSMA_ApplicationShutdown" {
            # "This is a JSMA-Reserved jMsg"
            n76 = call-poly <userlib>:"JET_QSM - Add State(s).vi"("Jet_QSM refnum"=w218, "error in (no error)"=w214, "state(s)"="VI Exit") -> ("error out"=w217:errorcluster)  [unwired: 8 in]
          }
          frame "------ Actions  ------" {
            # "This is a section header; the state is never expected to execute"
          }
          frame "Accounts List: Update" {
            n77 = Unbundle By Name(w226) -> ("Accounts"=w224:refnum<class "UITable.lvclass">, "Accounts"=w225:refnum<class "AAccount.lvclass">[])
            n78 = for {
              tunnel: w225 -> [w230] mode=indexing
              tunnel: [w228] -> w223 mode=indexing
              n79 = call-dynamic "Get Info.vi"("AAccount in"=w230) -> ("Account Information"=w229:T3)  [unwired: 8 in, 2 out]
              n80 = call "Cluster to String Array.vi"("Account Information"=w229) -> ("Array"=w228:string[])
            }
            n81 = call-dynamic "UITable - Data Update.vi"("UITable Data"=w223, "UITable"=w224) -> ("UITable"=w221:refnum<class "UITable.lvclass">)  [unwired: 6 in, 3 out]
            n82 = Bundle By Name(cluster=w226, "Accounts"=w221) -> (w222:refnum<class "Module_UI_TopLevel.lvclass">)
          }
          frame "------ Window and Panel Control ------" {
            # "This is a section header; the state is never expected to execute"
          }
          frame "Window: Open" {
            # "This state is called to open the Window, if desired - By convention,. we always controls windows dynamically - NEVER using the VI Appearance Properties (they should be set to default)"
            n83 = call-dynamic "PanelOpen.vi"("JETPanel in"=w240) -> ("error out"=w235:errorcluster, "JETPanel out"=w234:refnum<class "JETPanel.lvclass">)  [unwired: 9 in]
            n84 = call <userlib>:"Set Window Title.vi"("error in (no error)"=w235, "Window Title"=w233, "JETPanel in"=w234) -> ()  [unwired: 7 in, 2 out]
            n85 = call-poly <userlib>:"JET_QSM - Add State(s).vi"("Jet_QSM refnum"=w238, "error in (no error)"=w237, "state(s)"="Control Update") -> ("error out"=w236:errorcluster)  [unwired: 8 in]
          }
          frame "Window: Close" {
            # "This state is called to close the Window, if desired - By convention,. we always controls windows dynamically - NEVER using the VI Appearance Properties"
            n86 = call-dynamic "PanelClose.vi"("JETPanel"=w246) -> ()  [unwired: 9 in, 2 out]
            n87 = call-poly <userlib>:"JET_QSM - Add State(s).vi"("Jet_QSM refnum"=w244, "error in (no error)"=w243, "state(s)"="Control Update") -> ("error out"=w242:errorcluster)  [unwired: 8 in]
          }
          frame "Control Update" {
            # "Update all control properties values from the status cluster in this state - in this way we can separate the View from the Model and Controller, as well as consolidate/reduce locals and property nodes"
            n88 = Unbundle By Name(w266) -> ("Account Number"=w265:string, "Routing Number"=w264:string, "Balance"=w263:dbl, "Interest Rate"=w262:dbl, "Interest Interval"=w261:u32, "Account Type"=w260:T1, "Limit"=w249:dbl, "Credit Interval"=w248:u32)
            n89 = call-poly <userlib>:"JET_QSM - Add State(s).vi"("Jet_QSM refnum"=w271, "error in (no error)"=w270, "state(s)"="Indicator Update") -> ("error out"=w269:errorcluster)  [unwired: 8 in]
            n90 = in-place {
              n91 = in-place-cluster #2(w266) -> ("Accounts"=w276:refnum<class "UITable.lvclass">)
              n92 = call <userlib>:"UITable - Filter Sort Display.vi"("UITable"=w276) -> ("UITable"=w275:refnum<class "UITable.lvclass">)  [unwired: 6 in, 4 out]
              n93 = in-place-cluster #2("Accounts"=w275) -> (w267:refnum<class "Module_UI_TopLevel.lvclass">)
            }
            n94 = local write "Account Number"(w265) -> ()
            n95 = local write "Routing Number"(w264) -> ()
            n96 = local write "Initial Balance"(w263) -> ()
            n97 = local write "Interest Rate"(w262) -> ()
            n98 = local write "Interest Interval (s)"(w261) -> ()
            n99 = local write "Credit Limit Interval (s)"(w248) -> ()
            n100 = local write "Credit Limit"(w249) -> ()
            n101 = case shown="\"Credit\"" w260 {
              tunnel: [_ w273 _] -> w256
              tunnel: [_ w273 _] -> w255
              tunnel: [w272 _ TRUE] -> w254
              tunnel: [w272 w273 _] -> w251
              tunnel: [w272 w273 _] -> w250
              frame "Savings", Default {
                w272 = TRUE
              }
              frame "Checking" {
                w273 = TRUE
              }
              frame "Credit" {
              }
            }
            n102 = call <userlib>:"VI Control - Disable Control.vi"("Disable? (T)"=w256) -> ("Disabled Attribute"=w259:T9)  [unwired: 7 in, 1 out]
            n103 = call <userlib>:"VI Control - Disable Control.vi"("Disable? (T)"=w255) -> ("Disabled Attribute"=w258:T9)  [unwired: 7 in, 1 out]
            n104 = call <userlib>:"VI Control - Disable Control.vi"("Disable? (T)"=w254) -> ("Disabled Attribute"=w257:T9)  [unwired: 7 in, 1 out]
            n105 = call <userlib>:"VI Control - Disable Control.vi"("Disable? (T)"=w251) -> ("Disabled Attribute"=w252:T9)  [unwired: 7 in, 1 out]
            n106 = call <userlib>:"VI Control - Disable Control.vi"("Disable? (T)"=w250) -> ("Disabled Attribute"=w253:T9)  [unwired: 7 in, 1 out]
            n107 = property on="Interest Rate" class="DigNum (strict)"("DisabledEnum"=w259) -> ()  [unwired: 2 in, 2 out]
            n108 = property on="Interest Interval (s)" class="DigNum (strict)"("DisabledEnum"=w258) -> ()  [unwired: 2 in, 2 out]
            n109 = property on="Routing Number" class="Str"("DisabledEnum"=w257) -> ()  [unwired: 2 in, 2 out]
            n110 = property on="Credit Limit" class="DigNum (strict)"("DisabledEnum"=w252) -> ()  [unwired: 2 in, 2 out]
            n111 = property on="Credit Limit Interval (s)" class="DigNum (strict)"("DisabledEnum"=w253) -> ()  [unwired: 2 in, 2 out]
          }
          frame "Indicator Update" {
            # "Update all indicator properties and values from the status cluster in this state - in this way we can separate the View from the Model and Controller, as well as consolidate/reduce property nodes"
          }
        }
      }
    }
    frame Error {
    }
  }
  "error out" <- w3
